vi "Test_connection.vi"() -> ()   [LabVIEW 2016]
uses:
  Instrument_Setup.vi
panel:
  out "String":string
  in  "error in":T1
  out "Instrument Responded?":bool
  out "error out":T1
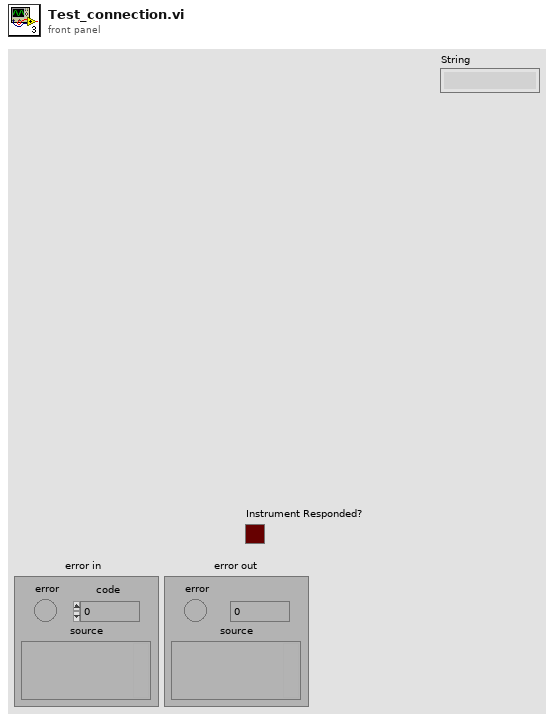
[diagram p1: front panel]
types:
  T1 = cluster{"error":bool, "code":i32, "source":string}
  T2 = cluster{"connection ID":refnum<k5>, "IP":string, "TCP Port":i32}
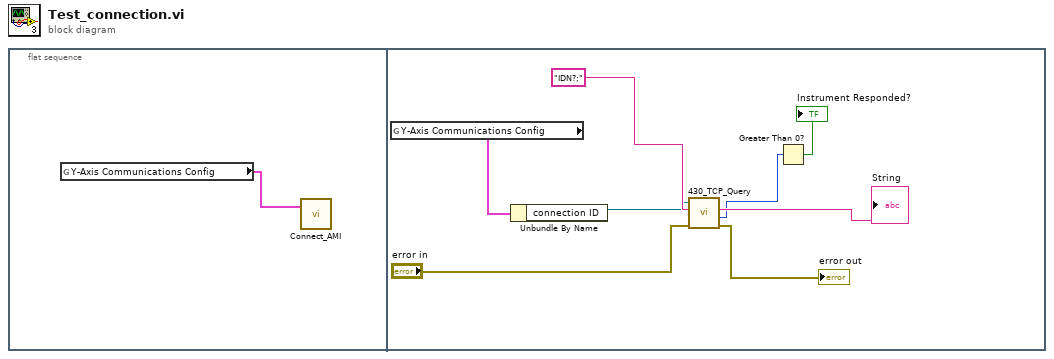
[diagram p0: block diagram]
diagram:
  n1 = flat-sequence {
    frame #0 {
      n2 = global read "Instrument_Setup.vi" "Y-Axis Communications Config"() -> (w1:T2)
      n3 = call "Connect_AMI.vi"("Communications Config"=w1) -> ()  [unwired: 1 in, 1 out]
    }
    frame #1 {
      n4 = global read "Instrument_Setup.vi" "Y-Axis Communications Config"() -> (w2:T2)
      n5 = Unbundle By Name(w2) -> ("connection ID"=w4:refnum<k5>)
      n6 = call "430_TCP_Query.vi"("error in (no error)"="error in", "Command"="IDN?;", "connection ID"=w4) -> ("error out"=→"error out":errorcluster, "Bytes Read"=w8:i32, "Response"=→"String":string)  [unwired: 4 in, 2 out]
      n7 = Greater Than 0?(x=w8) -> (x > 0?=→"Instrument Responded?":bool)
    }
  }
